vi "data_dashboard_feed.vi"() -> ()   [LabVIEW 2011]
uses:
  Output - Cluster b2g1.ctl
panel:
  in  "stop":bool
  out "Fehler":errorcluster
  # "Data Dashboard Feed"
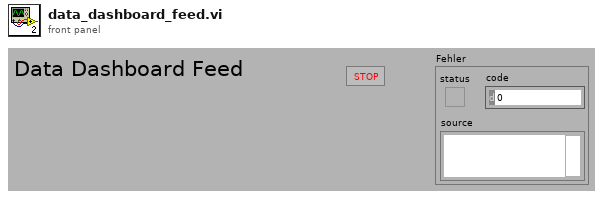
[diagram p1: front panel]
types:
  T1 = typedef "Output - Cluster b2g1.ctl" = cluster{"DFS-1 [dl]":u64, "FS-3 [l]":dbl, "DFS-1 [l/min]":dbl, "DS-1 [bar]":dbl, "V-10 ZU":bool, "V-14 ZU":bool, "FS-1 [l]":dbl, "FS-2 [l]":dbl, "TS-4 [°C]":dbl, "HS-1":bool, "V-13 [%]":u8, "V-15 [%]":u8, "P-4 [%]":u8, "P-5 [%]":u8, "Dosierung":bool, "MR Max Füllstand":bool, "MR Min Füllstand":bool, "Dosiermenge [l]":sgl, "V-14 AUF":bool, "V-10 AUF":bool, "T-1 Max Füllstand":bool, "T-1 Min Füllstand":bool, "T-2 Max Füllstand":bool, "T-2 Min Füllstand":bool, "pHS-1 [pH]":dbl, "P-4 RUN":bool, "P-5 RUN ":bool, "V-33 AUF":bool, "V-33 ZU":bool, "V-34 AUF":bool, "V-34 ZU":bool, "P-4 ERR":bool, "P-5 ERR":bool, "TS-5 [°C]":dbl, "TS-6 [°C]":dbl, "P-9 RUN":bool}
  T2 = enum32{"invalid app kind", "Development System", "Run Time System", "Student Edition", "Embedded LabVIEW", "Evaluation", "Custom"}
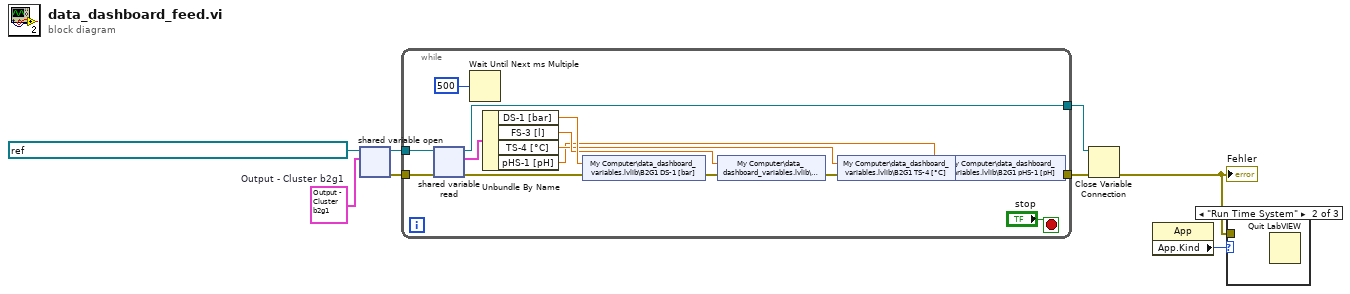
[diagram p0: block diagram]
diagram:
  w8 = T1 {"DFS-1 [dl]"=0, "FS-3 [l]"=0.0, "DFS-1 [l/min]"=0.0, "DS-1 [bar]"=0.0, "V-10 ZU"=FALSE, "V-14 ZU"=FALSE, "FS-1 [l]"=0.0, "FS-2 [l]"=0.0, "TS-4 [°C]"=0.0, "HS-1"=FALSE, "V-13 [%]"=0, "V-15 [%]"=0, "P-4 [%]"=0, "P-5 [%]"=0, "Dosierung"=FALSE, "MR Max Füllstand"=FALSE, "MR Min Füllstand"=FALSE, "Dosiermenge [l]"=0.0, "V-14 AUF"=FALSE, "V-10 AUF"=FALSE, "T-1 Max Füllstand"=FALSE, "T-1 Min Füllstand"=FALSE, "T-2 Max Füllstand"=FALSE, "T-2 Min Füllstand"=FALSE, "pHS-1 [pH]"=0.0, "P-4 RUN"=FALSE, "P-5 RUN "=FALSE, "V-33 AUF"=FALSE, "V-33 ZU"=FALSE, "V-34 AUF"=FALSE, "V-34 ZU"=FALSE, "P-4 ERR"=FALSE, "P-5 ERR"=FALSE, "TS-5 [°C]"=0.0, "TS-6 [°C]"=0.0, "P-9 RUN"=FALSE}  # Output - Cluster b2g1
  n1 = shared-variable-open(refnum<k21> "ni.var.psp://10.27.40.24/variables - b2g1/data - network - b2g1" ("output variable"), w8) -> (w3:refnum<k21>, w5:errorcluster)  [unwired: 2 in]
  n2 = while {
    tunnel: w5 -> [w23]
    tunnel: w3 -> [w22]
    tunnel: [w9] -> w2
    tunnel: [w16] -> w1
    stop <- "stop" stop-if-true
    n3 = shared-variable-read(w22, w23) -> (w16:refnum<k21>, w19:errorcluster, w21:T1)  [unwired: 1 out]
    n4 = Wait Until Next ms Multiple(millisecond multiple=u32 500) -> ()  [unwired: 1 out]
    n5 = Unbundle By Name(w21) -> ("DS-1 [bar]"=w20:dbl, "FS-3 [l]"=w15:dbl, "TS-4 [°C]"=w14:dbl, "pHS-1 [pH]"=w13:dbl)
    n6 = shared-variable "My Computer\\data_dashboard_variables.lvlib\\B2G1 DS-1 [bar]"(w20, error in=w19) -> (error out=w12:errorcluster)
    n7 = shared-variable "My Computer\\data_dashboard_variables.lvlib\\B2G1 FS-3 [l]"(w15, error in=w12) -> (error out=w11:errorcluster)
    n8 = shared-variable "My Computer\\data_dashboard_variables.lvlib\\B2G1 TS-4 [°C]"(w14, error in=w11) -> (error out=w10:errorcluster)
    n9 = shared-variable "My Computer\\data_dashboard_variables.lvlib\\B2G1 pHS-1 [pH]"(w13, error in=w10) -> (error out=w9:errorcluster)
  }
  n10 = Close Variable Connection(8:w2, 11:w1) -> (0:w4:errorcluster)
  "Fehler" <- w4
  n11 = property class="App"() -> ("App.Kind"=w6:T2)  [unwired: 2 in, 2 out]
  n12 = case shown="\"Run Time System\"" w6 {
    tunnel: w4 -> [_ _ _]
    frame "invalid app kind", Default {
    }
    frame "Run Time System" {
      n13 = Quit LabVIEW() -> ()  [unwired: 1 in]
    }
    frame "Development System" {
    }
  }
